vi "Read Configuration.vi"(8 "Error In":errorcluster, 11 "CS++RTWatchdogActor in":refnum<class "CS++RTWatchdogActor.lvclass">) -> (0 "Error Out":errorcluster, 3 "CS++RTWatchdogActor out":refnum<class "CS++RTWatchdogActor.lvclass">)   [LabVIEW 2016, in "CS++RTWatchdog.lvlib" / "CS++RTWatchdogActor.lvclass"]
doc: "Read watchdog configuration data."
uses:
  CS++RTWatchdogActor.lvclass
  CS++RTWatchdogActor.lvclass/CS++RTWatchdogActor.ctl
  CSPP_Core/Classes/CS++BaseClasses/Factory/CS++Factory.lvclass
  CSPP_Core/Libraries/Utilities/CS++Utilities.lvlib
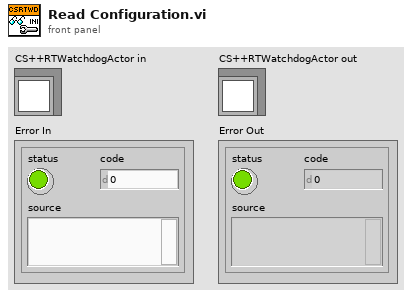
[diagram p1: front panel]
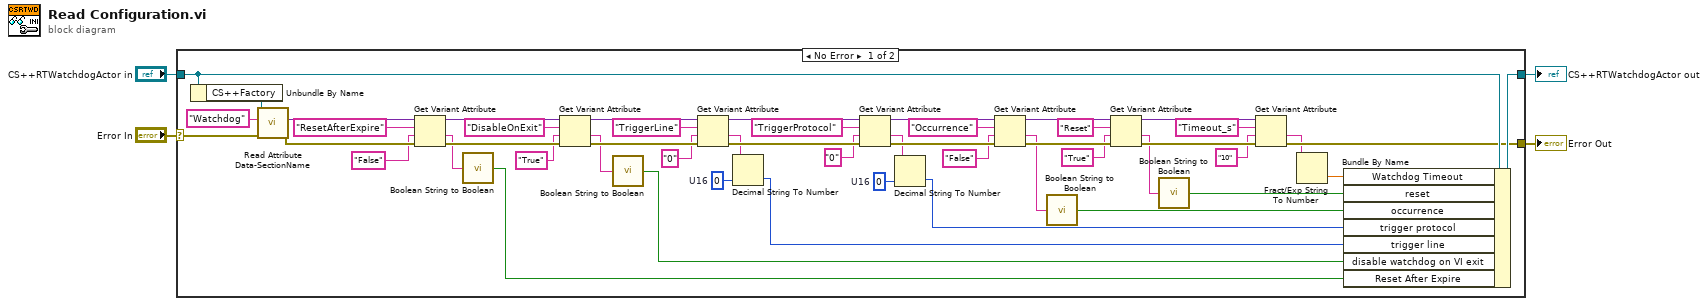
[diagram p0: block diagram]
diagram:
  n1 = case shown="No Error" "Error In" {
    selector: "Error In" -> [w36 w56]
    tunnel: [w28 w56] -> w3
    tunnel: [w39 w55] -> w1
    tunnel: "CS++RTWatchdogActor in" -> [w40 w55]
    frame No Error {
      w22 = u16 0  # U16
      w25 = u16 0  # U16
      n2 = Unbundle By Name(w40) -> ("CS++Factory"=w38:refnum<class "CS++Factory.lvclass">)
      n3 = call-dynamic "Read Attribute Data-SectionName.vi"("error in (no error)"=w36, "Object Name"="Watchdog" ("section"), "CS++Factory in"=w38) -> ("error out"=w34:errorcluster, "Attribute Data"=w35:variant)  [unwired: 6 in, 1 out]
      n4 = Get Variant Attribute(Variant=w35, name="ResetAfterExpire" ("key"), default value (empty Variant)="False" ("key"), error in=w34) -> (duplicate Variant=w32:variant, value=w15:string, error out=w31:errorcluster)  [unwired: 1 out]
      n5 = call "Boolean String to Boolean.vi"("T/F String"=w15) -> ("Value"=w14:bool)
      n6 = Get Variant Attribute(Variant=w32, name="DisableOnExit" ("key"), default value (empty Variant)="True" ("key"), error in=w31) -> (duplicate Variant=w30:variant, value=w12:string, error out=w53:errorcluster)  [unwired: 1 out]
      n7 = call "Boolean String to Boolean.vi"("T/F String"=w12) -> ("Value"=w11:bool)
      n8 = Get Variant Attribute(Variant=w30, name="TriggerLine" ("key"), default value (empty Variant)="0" ("key"), error in=w53) -> (duplicate Variant=w29:variant, value=w27:string, error out=w50:errorcluster)  [unwired: 1 out]
      n9 = Decimal String To Number(string=w27, default (0L)=w25) -> (number=w24:u16)  [unwired: 1 in, 1 out]
      n10 = Get Variant Attribute(Variant=w29, name="TriggerProtocol" ("key"), default value (empty Variant)="0" ("key"), error in=w50) -> (duplicate Variant=w48:variant, value=w21:string, error out=w47:errorcluster)  [unwired: 1 out]
      n11 = Decimal String To Number(string=w21, default (0L)=w22) -> (number=w20:u16)  [unwired: 1 in, 1 out]
      n12 = Get Variant Attribute(Variant=w48, name="Occurrence" ("key"), default value (empty Variant)="False" ("key"), error in=w47) -> (duplicate Variant=w45:variant, value=w9:string, error out=w44:errorcluster)  [unwired: 1 out]
      n13 = call "Boolean String to Boolean.vi"("T/F String"=w9) -> ("Value"=w8:bool)
      n14 = Get Variant Attribute(Variant=w45, name="Reset" ("key"), default value (empty Variant)="True" ("key"), error in=w44) -> (duplicate Variant=w42:variant, value=w6:string, error out=w41:errorcluster)  [unwired: 1 out]
      n15 = call "Boolean String to Boolean.vi"("T/F String"=w6) -> ("Value"=w5:bool)
      n16 = Get Variant Attribute(Variant=w42, name="Timeout_s" ("key"), default value (empty Variant)="10" ("key"), error in=w41) -> (value=w18:string, error out=w28:errorcluster)  [unwired: 2 out]
      n17 = Fract/Exp String To Number(string=w18) -> (number=w17:dbl)  [unwired: 3 in, 1 out]
      n18 = Bundle By Name(cluster=w40, "Watchdog Timeout"=w17, "reset"=w5, "occurrence"=w8, "trigger protocol"=w20, "trigger line"=w24, "disable watchdog on VI exit"=w11, "Reset After Expire"=w14) -> (w39:refnum<class "CS++RTWatchdogActor.lvclass">)
    }
    frame Error {
    }
  }
  "Error Out" <- w3
  "CS++RTWatchdogActor out" <- w1
